vi "CC Script Set Status Value.vi"(7 "Time Stamp":timestamp, 8 "error in (no error)":errorcluster, 9 "Value":dbl, 10 "Ch Name":string, 11 "Data Q":refnum<queue>) -> (0 "error out":errorcluster)   [LabVIEW 2024]
uses:
  Subsystems/SS cluster Data Queue type.ctl
  hk-channel-class/hk-channel-class/HK Item/HK Channel cluster Telemetry Data.ctl
  hk-channel-class/hk-channel-class/HK Item/HK Channel enum Data Type.ctl
  hk-channel-class/hk-channel-class/HK Item/HK Item.lvclass
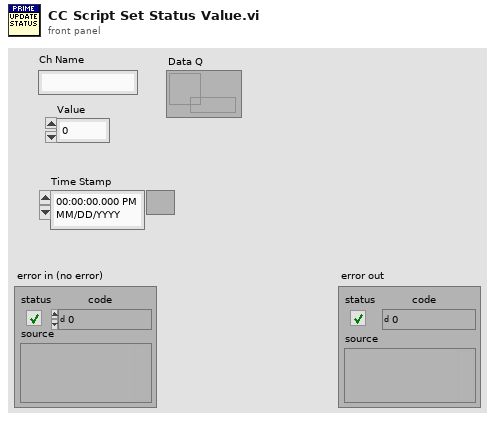
[diagram p1: front panel]
types:
  T1 = typedef "HK Item.lvclass/HK Channel enum Data Type.ctl" = enum16{"Floating Point", "Integer", "Enum", "String", "Waveform", "File"}
  T2 = typedef "HK Item.lvclass/HK Channel cluster Telemetry Data.ctl" = cluster{"Ch Names":string[], "Ch Values":dbl[], "Timestamp":timestamp, "Data Type":T1}
  T3 = typedef "SS cluster Data Queue type.ctl" = cluster{"Source":string, "Type":string, "Data":variant}
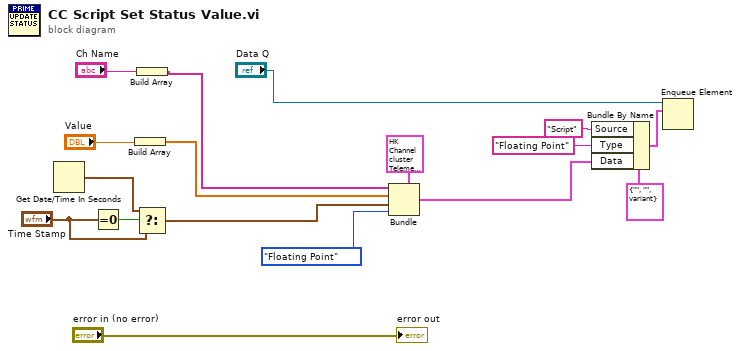
[diagram p0: block diagram]
diagram:
  n1 = Get Date/Time In Seconds() -> (seconds since 1Jan1904=w7:timestamp)
  n2 = Equal To 0?(x="Time Stamp") -> (x = 0?=w9:bool)
  n3 = Build Array("Value") -> (w1:dbl[])
  n4 = Build Array("Ch Name") -> (w3:string[])
  n5 = Select(t=w7, s=w9, f="Time Stamp") -> (s? t:f=w6:timestamp)
  n6 = Bundle(cluster=T2 {"Ch Names"=[], "Ch Values"=[], "Timestamp"=timestamp(0 s since 1904-01-01), "Data Type"=enum."Floating Point"}, "Ch Names"=w3, "Ch Values"=w1, "Timestamp"=w6, "Data Type"=HK_Channel_enum_Data_Type."Floating Point") -> (w12:T2)
  n7 = Bundle By Name(cluster=T3 {"Source"="", "Type"="", "Data"=variant} ("element"), "Source"="Script", "Type"="Floating Point" ("Data Type"), "Data"=w12) -> (w14:T3)
  n8 = Enqueue Element(queue="Data Q", element=w14) -> ()  [unwired: 2 in, 3 out]
  "error out" <- "error in (no error)"
